vi "Test Simple Connection.vi"() -> ()   [LabVIEW 2013]
uses:
  <vilib>/LabVIEW Open Source Project/MQTT Control Packets/Control Packets/CONNECT/CONNECT.lvclass
  <vilib>/LabVIEW Open Source Project/MQTT Control Packets/Control Packets/CONNACK/Connect Return Code -- enum.ctl
  MQTT_TCP/Connection/TCPConnection.lvclass
  <vilib>/LabVIEW Open Source Project/MQTT Control Packets/Control Packets/PUBLISH/PUBLISH.lvclass
  <vilib>/LabVIEW Open Source Project/MQTT Control Packets/Control Packets/ControlPacket/ControlPacket.lvclass
  Connection/Connection.lvclass
  <vilib>/LabVIEW Open Source Project/MQTT Control Packets/Control Packets/CONNACK/CONNACK.lvclass
  <vilib>/LabVIEW Open Source Project/MQTT Control Packets/Control Packets/ControlPacket/ControlPacket.lvclass/ControlPacket.ctl
  <vilib>/LabVIEW Open Source Project/MQTT Control Packets/Control Packets/DISCONNECT/DISCONNECT.lvclass
  <vilib>/LabVIEW Open Source Project/MQTT Control Packets/Control Packets/MQTT_311/MQTTVersion.lvclass
panel:
  in  "Range (max)":dbl=1.0
  out "randomNumber":dbl
  out "Topic":string
  out "connected":bool
  in  "Connect to Server":bool
  out "client":errorcluster
  out "server":errorcluster
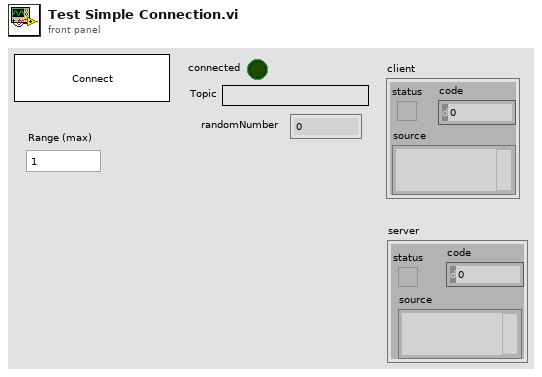
[diagram p1: front panel]
types:
  T1 = enum16{"Standard", "Buffered", "CRLF", "Immediate"}
  T2 = cluster{"Packet":refnum<class "ControlPacket.lvclass">, "Direction":enum16{"In", "Out"}}
  T3 = cluster{"connected":refnum<user-event>, "Incoming Message":refnum<user-event>}
  T4 = cluster{"Connection":refnum<class "TCPConnection.lvclass">, "Public Events":cluster{"connected":refnum<user-event>, "Incoming Message":refnum<user-event>}, "Payload":refnum<queue>}
  T5 = typedef "MQTT_Control_Packets.lvlib/CONNACK.lvclass/Connect Return Code -- enum.ctl" = enum16{"Connection accepted", "Unacceptable protocol version", "Identifier Rejected", "Server Unavailable", "Bad Username or Password", "Not Authorized"}
  T6 = typedef "MQTT_Control_Packets.lvlib/ControlPacket.lvclass/Control Packet Type -- enum.ctl" = enum16{"Reserved", "CONNECT", "CONNACK", "PUBLISH", "PUBACK", "PUBREC", "PUBREL", "PUBCOMP", "SUBSCRIBE", "SUBACK", "UNSUBSCRIBE", "UNSUBACK", "PINGREQ", "PINGRESP", "DISCONNECT", "AUTH"}
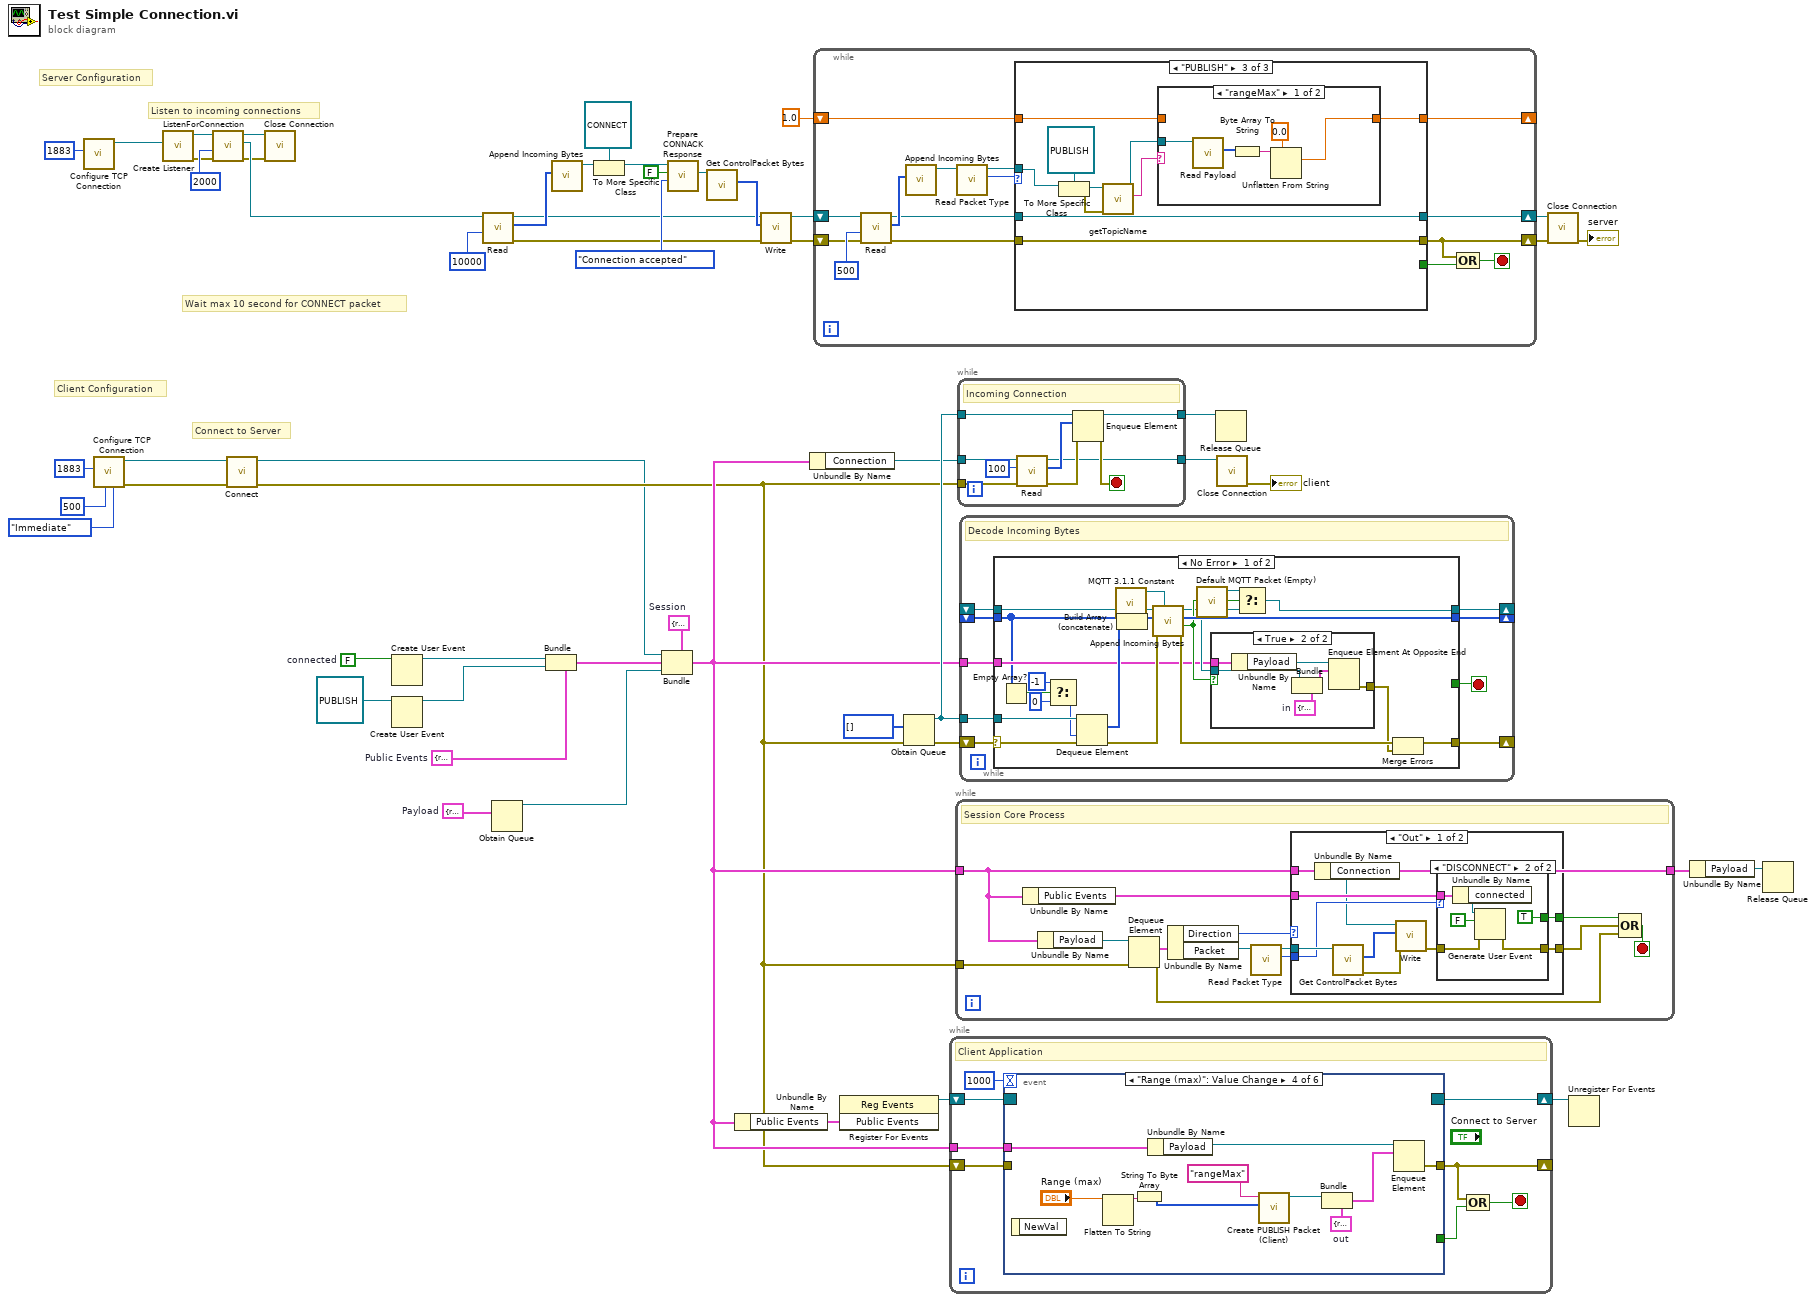
[diagram p0: block diagram]
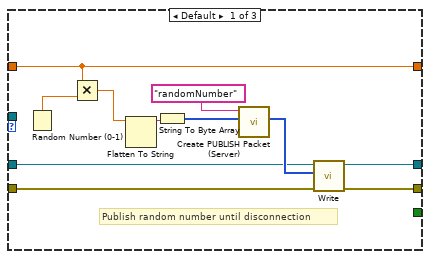
[diagram p2: hidden frame]
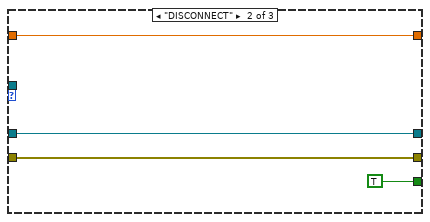
[diagram p3: hidden frame]
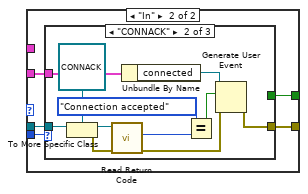
[diagram p6: hidden frame]
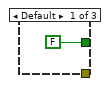
[diagram p7: hidden frame]
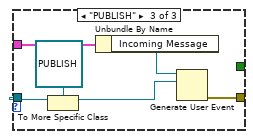
[diagram p8: hidden frame]
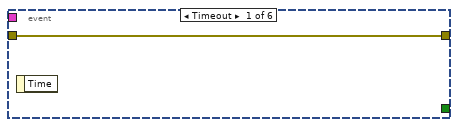
[diagram p9: hidden frame]
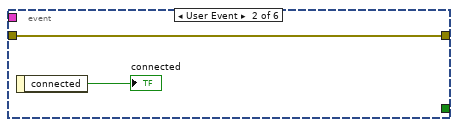
[diagram p10: hidden frame]
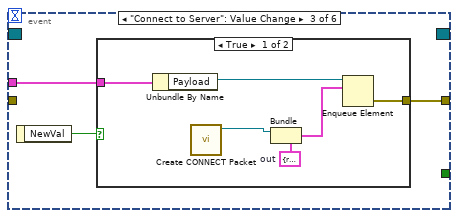
[diagram p11: hidden frame]
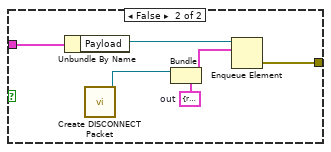
[diagram p12: hidden frame]
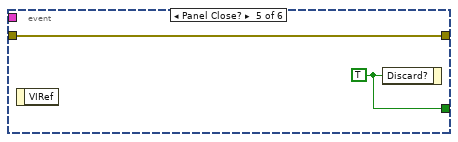
[diagram p13: hidden frame]
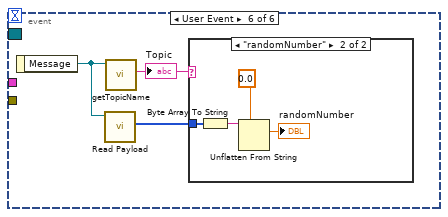
[diagram p14: hidden frame]
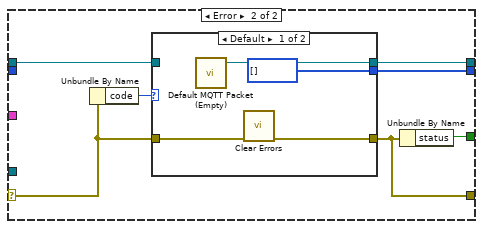
[diagram p17: hidden frame]
diagram:
  w25 = T2 {"Packet"=refnum, "Direction"=enum."In"}  # Payload
  w38 = T3 {"connected"=refnum, "Incoming Message"=refnum}  # Public Events
  w39 = FALSE  # connected
  w41 = T4 {"Connection"=refnum, "Public Events"={"connected"=refnum, "Incoming Message"=refnum}, "Payload"=refnum}  # Session
  # "Connect to Server"
  # "Client Configuration"
  # "Listen to incoming connections"
  # "Wait max 10 second for CONNECT packet"
  # "Server Configuration"
  n1 = call "Configure TCP Connection.vi"("remote port (80)"=u16 1883) -> ("TCPConnection"=w7:refnum<class "TCPConnection.lvclass">)  [unwired: 9 in, 1 out]
  n2 = call "Configure TCP Connection.vi"("Read Mode (Immediate)"=T1."Immediate" ("mode (standard)"), "timeout (100ms)"=500, "remote port (80)"=u16 1883) -> ("error out"=w9:errorcluster, "TCPConnection"=w13:refnum<class "TCPConnection.lvclass">)  [unwired: 7 in]
  n3 = call "Create Listener.vi"("Connection Configuration"=w7) -> ("error out"=w2:errorcluster, "Listener"=w6:refnum<class "Connection.lvclass">)  [unwired: 9 in]
  n4 = call "ListenForConnection.vi"("error in (no error)"=w2, "timeout (ms)"=2000 ("bytes to read (100)"), "Listener"=w6) -> ("error out"=w1:errorcluster, "Connection"=w3:refnum<class "Connection.lvclass">, "Listener out"=w4:refnum<class "Connection.lvclass">)  [unwired: 5 in, 1 out]
  n5 = call "Connect.vi"("error in (no error)"=w9, "Connection in"=w13) -> ("error out"=w11:errorcluster, "Connection out"=w10:refnum<class "TCPConnection.lvclass">)  [unwired: 8 in]
  n6 = call-dynamic "Close Connection.vi"("error in (no error)"=w1, "Connection in"=w4) -> ()  [unwired: 8 in, 2 out]
  n7 = Create User Event(user event datatype=w39) -> (user event=w40:refnum<user-event>)  [unwired: 1 in, 1 out]
  n8 = Create User Event(user event datatype=refnum<class "PUBLISH.lvclass"> refnum ("Message")) -> (user event=w30:refnum<user-event>)  [unwired: 1 in, 1 out]
  n9 = call "Read.vi"("timeout (1000 ms)"=10000 ("bytes to read (100)"), "TCPConnection in"=w3) -> ("error out"=w18:errorcluster, "Bytes"=w17:u8[], "TCPConnection out"=w16:refnum<class "Connection.lvclass">)  [unwired: 5 in, 2 out]
  n10 = Obtain Queue(element data type=w25) -> (queue out=w23:refnum<queue>)  [unwired: 4 in, 2 out]
  n11 = Bundle(cluster=w38, "connected"=w40, "Incoming Message"=w30) -> (w24:T3)
  n12 = call <vilib>:"Append Incoming Bytes.vi"("Incoming Packets"=w17) -> ("ControlPacket"=w54:refnum<class "ControlPacket.lvclass">)  [unwired: 7 in, 3 out]
  n13 = To More Specific Class(target class=refnum<class "CONNECT.lvclass"> refnum ("CONNECT in"), reference=w54) -> (specific class reference=w53:refnum<class "CONNECT.lvclass">)  [unwired: 1 in, 1 out]
  n14 = Bundle(cluster=w41, "Connection"=w10, "Public Events"=w24, "Payload"=w23) -> (w21:T4)
  n15 = call-dynamic "Prepare CONNACK Response.vi"("Return Code"=Connect_Return_Code_--_enum."Connection accepted", "Session Present"=FALSE, "CONNECT in"=w53) -> ("CONNACK response"=w50:refnum<class "CONNACK.lvclass">)  [unwired: 5 in, 3 out]
  n16 = call <vilib>:"Get ControlPacket Bytes.vi"("ControlPacket"=w50) -> ("Bytes Stream"=w51:u8[])  [unwired: 7 in, 3 out]
  n17 = Unbundle By Name(w21) -> ("Public Events"=w37:T3)
  n18 = call "Write.vi"("error in (no error)"=w18, "Bytes"=w51, "Connection in"=w16) -> ("error out"=w28:errorcluster, "Connection"=w29:refnum<class "Connection.lvclass">)  [unwired: 7 in]
  n19 = Unbundle By Name(w21) -> ("Connection"=w20:refnum<class "TCPConnection.lvclass">)
  n20 = while {
    shift-right: [w61] -> w27
    shift-left: w29 -> [w66]
    shift-right: [w58] -> w26
    shift-left: w28 -> [w65]
    shift-right: [w56] -> _
    shift-left: 1.0 -> [w57]
    stop <- w59 stop-if-true
    n21 = call "Read.vi"("error in (no error)"=w65, "timeout (1000 ms)"=500 ("bytes to read (100)"), "TCPConnection in"=w66) -> ("error out"=w62:errorcluster, "Bytes"=w69:u8[], "TCPConnection out"=w63:refnum<class "Connection.lvclass">)  [unwired: 4 in, 2 out]
    n22 = call <vilib>:"Append Incoming Bytes.vi"("Incoming Packets"=w69) -> ("ControlPacket"=w68:refnum<class "ControlPacket.lvclass">)  [unwired: 7 in, 3 out]
    n23 = call <vilib>:"Read Packet Type.vi"("ControlPacket in"=w68) -> ("Control Packet Type"=w64:T6, "ControlPacket out"=w55:refnum<class "ControlPacket.lvclass">)  [unwired: 9 in]
    n24 = case shown="\"PUBLISH\"" w64 {
      tunnel: w63 -> [w76 w84 w94]
      tunnel: w62 -> [w73 w83 w93]
      tunnel: [w75 w84 w94] -> w61
      tunnel: [w74 w83 w93] -> w58
      tunnel: [_ TRUE _] -> w60
      tunnel: w57 -> [w70 w81 w87]
      tunnel: [w70 w81 w86] -> w56
      tunnel: w55 -> [_ _ w91]
      frame Default {
        # "Publish random number until disconnection"
        n25 = Random Number (0-1)() -> (number: 0 to 1=w72:dbl)
        n26 = Multiply(x=w70, y=w72) -> (x*y=w71:dbl)
        n27 = Flatten To String(anything=w71) -> (data string=w78:string)  [unwired: 3 in, 2 out]
        n28 = String To Byte Array(string=w78) -> (unsigned byte array=w79:u8[])
        n29 = call <vilib>:"Create PUBLISH Packet (Server).vi"("Payload"=w79, "Topic Name"="randomNumber") -> ("Bytes Stream"=w80:u8[])  [unwired: 6 in, 3 out]
        n30 = call "Write.vi"("error in (no error)"=w73, "Bytes"=w80, "Connection in"=w76) -> ("error out"=w74:errorcluster, "Connection"=w75:refnum<class "Connection.lvclass">)  [unwired: 7 in]
      }
      frame "DISCONNECT" {
      }
      frame "PUBLISH" {
        n31 = To More Specific Class(target class=refnum<class "PUBLISH.lvclass"> refnum ("event data"), reference=w91) -> (specific class reference=w89:refnum<class "PUBLISH.lvclass">, error out=w90:errorcluster)  [unwired: 1 in]
        n32 = call <vilib>:"getTopicName.vi"("error in (no error)"=w90, "PUBLISH in"=w89) -> ("Topic"=w88:string, "PUBLISH out"=w85:refnum<class "PUBLISH.lvclass">)  [unwired: 7 in, 1 out]
        n33 = case shown="\"rangeMax\"" w88 {
          tunnel: w87 -> [_ w100]
          tunnel: [w95 w100] -> w86
          tunnel: w85 -> [w99 _]
          frame "rangeMax" {
            n34 = call <vilib>:"Read Payload.vi"("ControlPacket in"=w99) -> ("Payload"=w96:u8[])  [unwired: 9 in, 1 out]
            n35 = Byte Array To String(unsigned byte array=w96) -> (string=w97:string)
            n36 = Unflatten From String(type=0.0, binary string=w97) -> (value=w95:dbl)  [unwired: 3 in, 2 out]
          }
          frame Default {
          }
        }
      }
    }
    n37 = Compound Arithmetic op=OR(w58, w60) -> (w59:bool)
  }
  n38 = register-events(w37) -> (reference out=w43:refnum<event-registration>)  [unwired: 2 in, 1 out]
  n39 = Obtain Queue(element data type=u8[] [] ("Remaining Packets"), error in (no error)=w11) -> (queue out=w47:refnum<queue>, error out=w45:errorcluster)  [unwired: 3 in, 1 out]
  n40 = while {
    shift-right: [w106] -> w42
    shift-left: w43 -> [w107]
    shift-right: [w104] -> _
    shift-left: w11 -> [w105]
    tunnel: w21 -> [w102]
    stop <- w103 stop-if-true
    # "Client Application"
    n41 = event shown="[3] \"Range (max)\": Value Change" {
      selector: w107 -> [_ _ _ _ _ _]
      dyn-events: [_ _ _ _ _ _] -> w106
      timeout: 1000 -> [_ _ _ _ _ _]
      tunnel: [_ _ _ _ w138 _] -> w101
      tunnel: [w109 w111 w112 w135 w137 _] -> w104
      tunnel: w105 -> [w109 w111 _ _ w137 _]
      tunnel: w102 -> [_ _ w113 w136 _ _]
      event Timeout {
        n42 = event-data() -> ()  [unwired: 1 in, 1 out]
      }
      event User Event {
        n43 = event-data() -> ("connected"=→"connected":bool)  [unwired: 1 in]
      }
      event "Connect to Server": Value Change {
        n44 = event-data() -> ("NewVal"=w114:bool)  [unwired: 1 in]
        n45 = case shown="True" w114 {
          tunnel: w113 -> [w120 w126]
          tunnel: [w118 w124] -> w112
          frame True {
            w117 = T2 {"Packet"=refnum, "Direction"=enum."Out"}  # out
            n46 = Unbundle By Name(w120) -> ("Payload"=w119:refnum<queue>)
            n47 = call <vilib>:"Create CONNECT Packet.vi"() -> ("CONNECT"=w116:refnum<class "CONNECT.lvclass">)  [unwired: 9 in, 2 out]
            n48 = Bundle(cluster=w117, "Packet"=w116) -> (w115:T2)  [unwired: 1 in]
            n49 = Enqueue Element(queue=w119, element=w115) -> (error out=w118:errorcluster)  [unwired: 2 in, 2 out]
          }
          frame False {
            w121 = T2 {"Packet"=refnum, "Direction"=enum."Out"}  # out
            n50 = Unbundle By Name(w126) -> ("Payload"=w125:refnum<queue>)
            n51 = call <vilib>:"Create DISCONNECT Packet.vi"() -> ("DISCONNECT"=w123:refnum<class "DISCONNECT.lvclass">)  [unwired: 9 in, 2 out]
            n52 = Bundle(cluster=w121, "Packet"=w123) -> (w122:T2)  [unwired: 1 in]
            n53 = Enqueue Element(queue=w125, element=w122) -> (error out=w124:errorcluster)  [unwired: 2 in, 2 out]
          }
        }
      }
      event "Range (max)": Value Change {
        w133 = T2 {"Packet"=refnum, "Direction"=enum."Out"}  # out
        n54 = event-data() -> ()  [unwired: 1 in, 1 out]
        n55 = Flatten To String(anything="Range (max)") -> (data string=w129:string)  [unwired: 3 in, 2 out]
        n56 = String To Byte Array(string=w129) -> (unsigned byte array=w128:u8[])
        n57 = Unbundle By Name(w136) -> ("Payload"=w134:refnum<queue>)
        n58 = call <vilib>:"Create PUBLISH Packet (Client).vi"("Payload"=w128, "Topic Name"="rangeMax") -> ("PUBLISH"=w131:refnum<class "PUBLISH.lvclass">)  [unwired: 6 in, 3 out]
        n59 = Bundle(cluster=w133, "Packet"=w131) -> (w132:T2)  [unwired: 1 in]
        n60 = Enqueue Element(queue=w134, element=w132) -> (error out=w135:errorcluster)  [unwired: 2 in, 2 out]
      }
      event Panel Close? {
        w138 = TRUE ("Discard?")
        n61 = event-data() -> ()  [unwired: 1 in, 1 out]
        n62 = event-data("Discard?"=w138) -> ()  [unwired: 1 in, 1 out]
      }
      event User Event {
        n63 = event-data() -> ("Message"=w141:refnum<class "PUBLISH.lvclass">)  [unwired: 1 in]
        n64 = call <vilib>:"Read Payload.vi"("ControlPacket in"=w141) -> ("Payload"=w139:u8[])  [unwired: 9 in, 1 out]
        n65 = call <vilib>:"getTopicName.vi"("PUBLISH in"=w141) -> ("Topic"=w140:string)  [unwired: 8 in, 2 out]
        "Topic" <- w140
        n66 = case shown="\"randomNumber\"" w140 {
          tunnel: w139 -> [_ w144]
          frame "False", Default {
          }
          frame "randomNumber" {
            n67 = Byte Array To String(unsigned byte array=w144) -> (string=w143:string)
            n68 = Unflatten From String(type=0.0, binary string=w143) -> (value=→"randomNumber":dbl)  [unwired: 3 in, 2 out]
          }
        }
      }
    }
    n69 = Compound Arithmetic op=OR(w104, w101) -> (w103:bool)
  }
  n70 = while {
    tunnel: w21 -> [w147]
    tunnel: [w147] -> w36
    tunnel: w11 -> [w156]
    stop <- w152 stop-if-true
    # "Session Core Process"
    n71 = Unbundle By Name(w147) -> ("Public Events"=w146:T3)
    n72 = Unbundle By Name(w147) -> ("Payload"=w151:refnum<queue>)
    n73 = Dequeue Element(queue=w151, error in (no error)=w156) -> (element=w150:T2, error out=w153:errorcluster)  [unwired: 1 in, 2 out]
    n74 = Unbundle By Name(w150) -> ("Direction"=w148:enum16{"In", "Out"}, "Packet"=w149:refnum<class "ControlPacket.lvclass">)
    n75 = call <vilib>:"Read Packet Type.vi"("ControlPacket in"=w149) -> ("Control Packet Type"=w158:T6, "ControlPacket out"=w157:refnum<class "ControlPacket.lvclass">)  [unwired: 9 in]
    n76 = case shown="\"Out\"" w148 {
      tunnel: w158 -> [w164 w180]
      tunnel: w157 -> [w166 w179]
      tunnel: [w168 w178] -> w155
      tunnel: [w167 w177] -> w154
      tunnel: w147 -> [w165 _]
      tunnel: w146 -> [w163 w176]
      frame "Out" {
        n77 = Unbundle By Name(w165) -> ("Connection"=w162:refnum<class "TCPConnection.lvclass">)
        n78 = call <vilib>:"Get ControlPacket Bytes.vi"("ControlPacket"=w166) -> ("error out"=w160:errorcluster, "Bytes Stream"=w161:u8[])  [unwired: 7 in, 2 out]
        n79 = call "Write.vi"("error in (no error)"=w160, "Bytes"=w161, "Connection in"=w162) -> ("error out"=w159:errorcluster)  [unwired: 7 in, 1 out]
        n80 = case shown="\"DISCONNECT\"" w164 {
          tunnel: [_ TRUE] -> w168
          tunnel: [w169 w173] -> w167
          tunnel: w159 -> [w169 w172]
          tunnel: w163 -> [_ w171]
          frame Default {
          }
          frame "DISCONNECT" {
            n81 = Unbundle By Name(w171) -> ("connected"=w170:refnum<user-event>)
            n82 = Generate User Event(user event=w170, event data cluster=FALSE ("event data"), error in=w172) -> (error out=w173:errorcluster)  [unwired: 1 in, 1 out]
          }
        }
      }
      frame "In" {
        n83 = case shown="\"CONNACK\"" w180 {
          tunnel: w179 -> [_ w192 w197]
          tunnel: [_ w187 w198] -> w177
          tunnel: [FALSE _ _] -> w178
          tunnel: w176 -> [_ w182 w194]
          frame Default {
          }
          frame "CONNACK" {
            n84 = To More Specific Class(target class=refnum<class "CONNACK.lvclass"> refnum ("CONNACK in"), reference=w192) -> (specific class reference=w190:refnum<class "CONNACK.lvclass">, error out=w185:errorcluster)  [unwired: 1 in]
            n85 = call <vilib>:"Read Return Code.vi"("error in (no error)"=w185, "CONNACK in"=w190) -> ("error out"=w186:errorcluster, "Return Code"=w189:T5)  [unwired: 7 in, 1 out]
            n86 = Unbundle By Name(w182) -> ("connected"=w183:refnum<user-event>)
            n87 = Equal?(x=Connect_Return_Code_--_enum."Connection accepted", y=w189) -> (x = y?=w188:bool)
            n88 = Generate User Event(user event=w183, event data cluster=w188, error in=w186) -> (error out=w187:errorcluster)  [unwired: 1 in, 1 out]
          }
          frame "PUBLISH" {
            n89 = To More Specific Class(target class=refnum<class "PUBLISH.lvclass"> refnum ("event data"), reference=w197) -> (specific class reference=w195:refnum<class "PUBLISH.lvclass">)  [unwired: 1 in, 1 out]
            n90 = Unbundle By Name(w194) -> ("Incoming Message"=w193:refnum<user-event>)
            n91 = Generate User Event(user event=w193, event data cluster=w195) -> (error out=w198:errorcluster)  [unwired: 2 in, 1 out]
          }
        }
      }
    }
    n92 = Compound Arithmetic op=OR(w155, w154, w153) -> (w152:bool)
  }
  n93 = while {
    tunnel: w47 -> [w207]
    tunnel: w20 -> [w204]
    tunnel: [w199] -> w44
    tunnel: [w206] -> w34
    tunnel: w11 -> [w202]
    stop <- w205 stop-if-true
    # "Incoming Connection"
    n94 = call "Read.vi"("error in (no error)"=w202, "bytes to read (100)"=100, "TCPConnection in"=w204) -> ("error out"=w201:errorcluster, "Bytes"=w200:u8[], "TCPConnection out"=w199:refnum<class "TCPConnection.lvclass">)  [unwired: 4 in, 2 out]
    n95 = Enqueue Element(queue=w207, element=w200, error in (no error)=w201) -> (queue out=w206:refnum<queue>, error out=w205:errorcluster)  [unwired: 1 in, 1 out]
  }
  n96 = while {
    shift-right: [w214] -> _
    shift-left: _ -> [w213]
    shift-right: [w212] -> _
    shift-left: w45 -> [w211]
    shift-right: [w215] -> _
    shift-left: _ -> [w216]
    tunnel: w21 -> [w208]
    tunnel: w47 -> [w209]
    stop <- w210 stop-if-true
    # "Decode Incoming Bytes"
    n97 = case shown="No Error" w211 {
      selector: w211 -> [w231 w248]
      tunnel: w216 -> [w237 w246]
      tunnel: [w227 w250] -> w215
      tunnel: [w235 w249] -> w214
      tunnel: w213 -> [w218 _]
      tunnel: [w228 w245] -> w212
      tunnel: [_ w244] -> w210
      tunnel: w209 -> [w234 _]
      tunnel: w208 -> [w222 _]
      frame No Error {
        # "No Error"
        n98 = Empty Array?(array=w218) -> (empty?=w221:bool)
        n99 = Select(t=-1 ("timeout in ms (-1)"), s=w221, f=0) -> (s? t:f=w217:i32)
        n100 = Dequeue Element(queue=w234, timeout in ms (-1)=w217, error in (no error)=w231) -> (element=w233:u8[], error out=w230:errorcluster)  [unwired: 2 out]
        n101 = call <vilib>:"MQTT 3.1.1 Constant.vi"() -> ("MQTT 3.1.1"=w236:refnum<class "MQTTVersion.lvclass">)  [unwired: 11 in]
        n102 = Build Array (concatenate)(w218, w233) -> (w232:u8[])
        n103 = call <vilib>:"Append Incoming Bytes.vi"("MQTT Version (3.1.1)"=w236, "error in (no error)"=w230, "Incoming Packets"=w232, "Incomplete ControlPacket"=w237) -> ("error out"=w229:errorcluster, "Complete Packet"=w225:bool, "Remaining Packets"=w235:u8[], "ControlPacket"=w224:refnum<class "ControlPacket.lvclass">)  [unwired: 4 in]
        n104 = call <vilib>:"Default MQTT Packet (Empty).vi"() -> ("No Packet"=w226:refnum<class "ControlPacket.lvclass">)  [unwired: 11 in]
        n105 = case shown="True" w225 {
          tunnel: [_ w243] -> w223
          tunnel: w224 -> [_ w240]
          tunnel: w222 -> [_ w238]
          frame False {
            # "No Packet received"
          }
          frame True {
            w242 = T2 {"Packet"=refnum, "Direction"=enum."In"}  # in
            # "Packet Received"
            n106 = Unbundle By Name(w238) -> ("Payload"=w239:refnum<queue>)
            n107 = Bundle(cluster=w242, "Packet"=w240) -> (w241:T2)  [unwired: 1 in]
            n108 = Enqueue Element At Opposite End(queue=w239, element=w241) -> (error out=w243:errorcluster)  [unwired: 2 in, 2 out]
          }
        }
        n109 = Select(t=w226, s=w225, f=w224) -> (s? t:f=w227:refnum<class "ControlPacket.lvclass">)
        n110 = Merge Errors(w229, w223) -> (w228:errorcluster)
      }
      frame Error {
        # "Handle Error"
        n111 = Unbundle By Name(w248) -> ("code"=w247:i32)
        n112 = case shown="Default" w247 {
          tunnel: [w251 w256] -> w250
          tunnel: w248 -> [w254 w255]
          tunnel: [w253 w255] -> w245
          tunnel: [u8[] [] ("Remaining Packets") _] -> w249
          tunnel: w246 -> [_ w256]
          frame Default {
            # "Malformed Packet"
            n113 = call <vilib>:"Default MQTT Packet (Empty).vi"() -> ("No Packet"=w251:refnum<class "ControlPacket.lvclass">)  [unwired: 11 in]
            n114 = call <vilib>:"Clear Errors.vi"("error in (no error)"=w254) -> ("error out"=w253:errorcluster)  [unwired: 6 in]
          }
          frame 1, 66, 1556 {
          }
        }
        n115 = Unbundle By Name(w245) -> ("status"=w244:bool)
      }
    }
  }
  n116 = Release Queue(queue=w34) -> ()  [unwired: 2 in, 3 out]
  n117 = call-dynamic "Close Connection.vi"("Connection in"=w44) -> ("error out"=→"client":errorcluster)  [unwired: 9 in, 1 out]
  n118 = call-dynamic "Close Connection.vi"("error in (no error)"=w26, "Connection in"=w27) -> ("error out"=→"server":errorcluster)  [unwired: 8 in, 1 out]
  n119 = Unregister For Events(event registration refnum=w42) -> ()  [unwired: 1 in, 1 out]
  n120 = Unbundle By Name(w36) -> ("Payload"=w35:refnum<queue>)
  n121 = Release Queue(queue=w35) -> ()  [unwired: 2 in, 3 out]
